vi "RemoteControl.GlobalVariable.vi"() -> ()   [LabVIEW 2019, in "RemoteControl.lvlib" / "RemoteControl.lvclass"]
uses:
  RemoteControl.lvclass
  Typedefs/Message--Cluster.ctl
panel:
  out "Message (RESponse)":T1={"Command"="", "Data"=variant(string ""), "ID"=""}
  in  "Connections":i32
  out "Message (REQuest)":T1={"Command"="", "Data"=variant(string ""), "ID"=""}
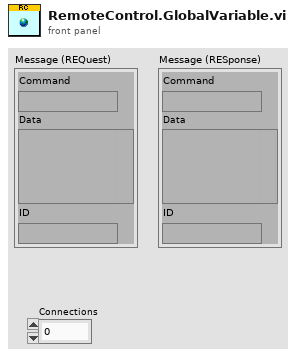
[diagram p1: front panel]
types:
  T1 = typedef "RemoteControl.lvlib/RemoteControl.lvclass/Message--Cluster.ctl" = cluster{"Command":string, "Data":variant, "ID":string}
diagram:
